vi "tx_prapare_transmit.vi"(8 "error in (no error)":errorcluster, 10 "input IQ waveform":cluster{"t0":dbl, "dt":dbl, "Y":cdb[]}={"t0"=0.0, "dt"=0.0, "Y"=array[6347 elements]}) -> (0 "error out":errorcluster, 2 "Scaled and Padded IQ waveform":cluster{"t0":dbl, "dt":dbl, "Y":cdb[]})   [LabVIEW 2012, in "gds_hw_config.lvlib"]
uses:
  gds_hw_config.lvlib
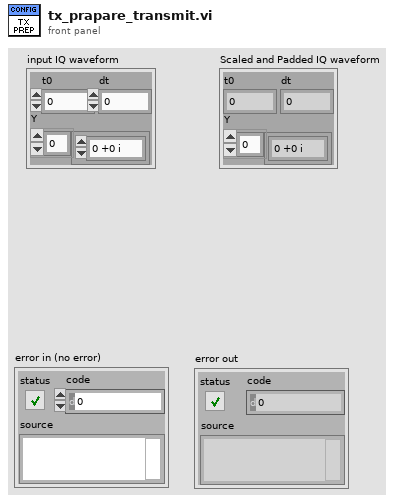
[diagram p1: front panel]
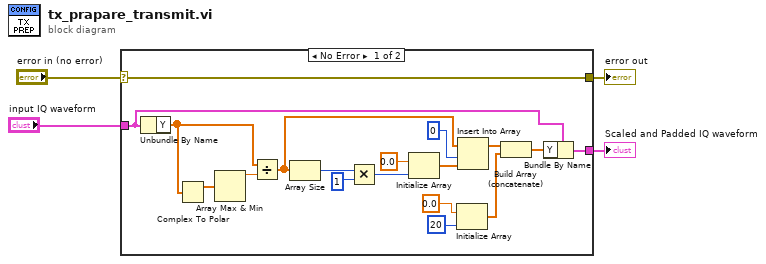
[diagram p0: block diagram]
diagram:
  n1 = case shown="No Error" "error in (no error)" {
    selector: "error in (no error)" -> [w20 w24]
    tunnel: [w20 w24] -> w3
    tunnel: [w21 w23] -> w2
    tunnel: "input IQ waveform" -> [w22 w23]
    frame No Error {
      n2 = Unbundle By Name(w22) -> ("Y"=w17:cdb[])
      n3 = Complex To Polar(r * e^(i*theta)=w17) -> (r=w19:dbl[])  [unwired: 1 out]
      n4 = Array Max & Min(array=w19) -> (max value=w18:dbl)  [unwired: 3 out]
      n5 = Divide(x=w17, y=w18) -> (x/y=w11:cdb[])
      n6 = Array Size(array=w11) -> (size(s)=w16:i32)
      n7 = Multiply(x=w16, y=1) -> (x*y=w14:i32)
      n8 = Initialize Array(0.0 ("element"), w14) -> (w12:dbl[])
      n9 = Initialize Array(0.0 ("element"), 20 ("dimension size")) -> (w7:dbl[])
      n10 = Insert Into Array(array=w11, index=0, new element=w12) -> (w6:cdb[])
      n11 = Build Array (concatenate)(w6, w7) -> (w5:cdb[])
      n12 = Bundle By Name(cluster=w22, "Y"=w5) -> (w21:cluster{"t0":dbl, "dt":dbl, "Y":cdb[]})
    }
    frame Error {
    }
  }
  "error out" <- w3
  "Scaled and Padded IQ waveform" <- w2
